vi "subGetListOfAllFilesToCheck.vi"(7 "Path to check blacklist":set{string}(c389), 11 "Path to Check":path) -> (3 "All Files in Dir":path[](array[path]))   [LabVIEW 2020, in "DependencyInspection.lvlib" / "CDependencyInspection.lvclass"]
uses:
  CDependencyInspection.lvclass
  <vilib>/Utility/LVLibp/NI_PackedLibraryUtility.lvlib
  <vilib>/regexp/Match Regular Expression.xnode
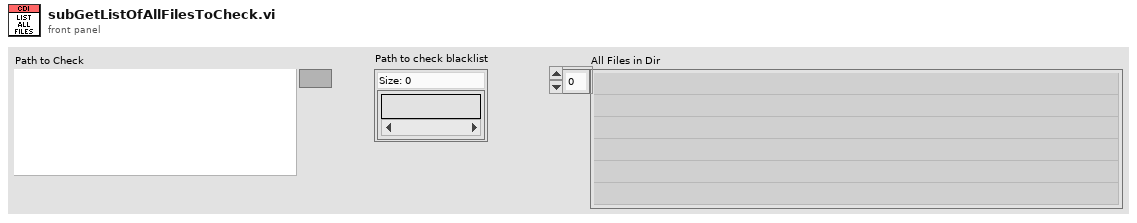
[diagram p1: front panel]
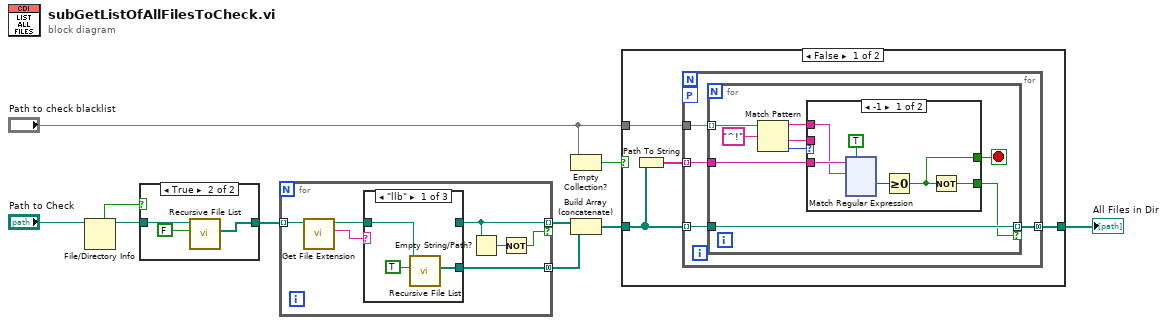
[diagram p0: block diagram]
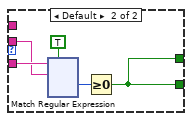
[diagram p2: hidden frame]
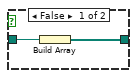
[diagram p4: hidden frame]
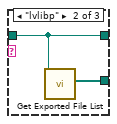
[diagram p5: hidden frame]
diagram:
  n1 = File/Directory Info(path="Path to Check") -> (path out=w9:path, directory=w10:bool)  [unwired: 1 in, 5 out]
  n2 = case shown="True" w10 {
    tunnel: [w12 w13] -> w5
    tunnel: w9 -> [w11 w15]
    frame False {
      n3 = Build Array(w11) -> (w12:path[])
    }
    frame True {
      n4 = call <vilib>:"Recursive File List.vi"("Treat LLBs as Folders?"=FALSE, "Folder Path"=w15) -> ("All Files in Dir"=w13:path[])  [unwired: 5 in, 4 out]
    }
  }
  n5 = for {
    tunnel: w5 -> [w20] mode=indexing
    tunnel: [w19] -> w7 mode=indexing if=w16
    tunnel: [w17] -> w6 mode=concatenating
    n6 = call <vilib>:"Get File Extension.vi"("file"=w20) -> ("lowercase file extension"=w21:string, "dup file"=w22:path)  [unwired: 6 in, 3 out]
    n7 = case shown="\"llb\"" w21 {
      tunnel: w22 -> [w25 w26 w28]
      tunnel: [w24 w27 _] -> w17
      tunnel: [_ w26 w28] -> w19
      frame "llb" {
        n8 = call <vilib>:"Recursive File List.vi"("Treat LLBs as Folders?"=TRUE, "Folder Path"=w25) -> ("All Files in Dir"=w24:path[])  [unwired: 5 in, 4 out]
      }
      frame "lvlibp" {
        n9 = call <vilib>:"Get Exported File List.vi"("packed library path"=w26) -> ("paths"=w27:path[])  [unwired: 8 in, 2 out]
      }
      frame Default {
      }
    }
    n10 = Empty String/Path?(string/path=w19) -> (empty?=w18:bool)
    n11 = Not(x=w18) -> (.not. x?=w16:bool)
  }
  n12 = Empty Collection?(1:"Path to check blacklist") -> (0:w3:bool)
  n13 = Build Array (concatenate)(w7, w6) -> (w2:path[])
  n14 = case shown="False" w3 {
    tunnel: "Path to check blacklist" -> [w32 _]
    tunnel: w2 -> [w31 w285]
    tunnel: [w29 w285] -> w1
    frame False {
      n15 = Path To String(path=w31) -> (string=w30:string[])
      n16 = for {
        tunnel: w32 -> [w36]
        tunnel: w31 -> [w34] mode=indexing
        tunnel: w30 -> [w35] mode=indexing
        workers-P: _ -> [_]
        tunnel: [w33] -> w29 mode=concatenating
        n17 = for {
          tunnel: w36 -> [w41] mode=indexing
          tunnel: w35 -> [w45]
          tunnel: w34 -> [w43]
          tunnel: [w43] -> w33 mode=indexing if=w42
          stop <- w44 stop-if-true
          n18 = Match Pattern(string=w41, regular expression="^!") -> (before substring=w37:string, after substring=w39:string, offset past match=w38:i32)  [unwired: 1 in, 1 out]
          n19 = case shown="-1" w38 {
            tunnel: w45 -> [w51 w170]
            tunnel: [w48 w166] -> w44
            tunnel: [w47 w166] -> w42
            tunnel: w39 -> [_ w167]
            tunnel: w37 -> [w46 _]
            frame -1 {
              n20 = xnode "Match Regular Expression"("input string"=w51, "regular expression"=w46, "ignore case? (F)"=TRUE) -> ("offset past match"=w49:i32)  [unwired: 3 in, 4 out]
              n21 = Greater Or Equal To 0?(x=w49) -> (x >= 0?=w48:bool)
              n22 = Not(x=w48) -> (.not. x?=w47:bool)
            }
            frame Default {
              n23 = xnode "Match Regular Expression"("input string"=w170, "regular expression"=w167, "ignore case? (F)"=TRUE) -> ("offset past match"=w168:i32)  [unwired: 3 in, 4 out]
              n24 = Greater Or Equal To 0?(x=w168) -> (x >= 0?=w166:bool)
            }
          }
        }
      }
    }
    frame True {
    }
  }
  "All Files in Dir" <- w1
